vi "Get Timestamp.vi"() -> (3 "result string":string)   [LabVIEW 2015]
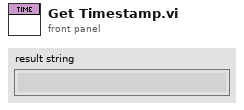
[diagram p1: front panel]
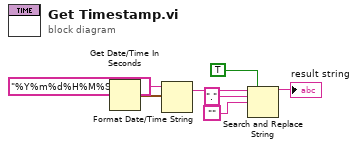
[diagram p0: block diagram]
diagram:
  n1 = Get Date/Time In Seconds() -> (seconds since 1Jan1904=w7:timestamp)
  n2 = Format Date/Time String(time format string (%c)="%Y%m%d%H%M%S%4u", seconds (now)=w7) -> (date/time string=w5:string)  [unwired: 1 in]
  n3 = Search and Replace String(replace all?=TRUE ("replace all? (F)"), input string=w5, search string="." ("regular expression (\"\")"), replace string="") -> (result string=→"result string":string)  [unwired: 4 in, 3 out]
